vi "resetOutput.vi"(8 "error in (no error)":errorcluster, 11 "K2602 in":refnum<class "K2602.lvclass">) -> (0 "error out":errorcluster, 3 "K2602 out":refnum<class "K2602.lvclass">)   [LabVIEW 2011, in "Hardware.lvlib" / "Channels.lvlib" / "K2602.lvclass"]
uses:
  K2602.lvclass
  AnalogOutput.lvclass
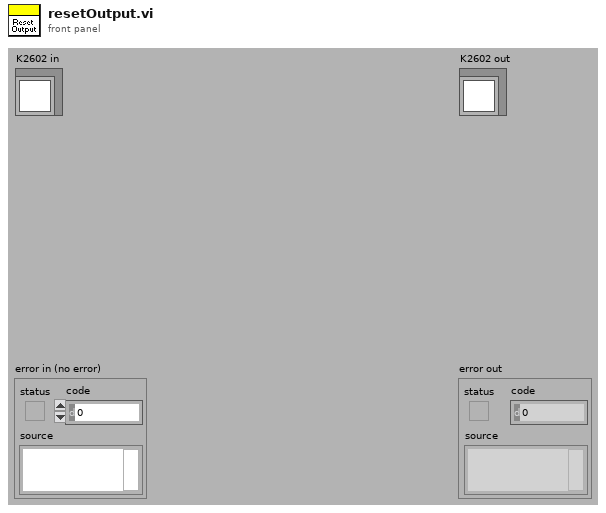
[diagram p1: front panel]
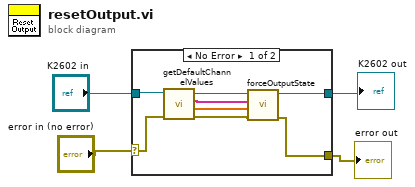
[diagram p0: block diagram]
diagram:
  n1 = case shown="No Error" "error in (no error)" {
    selector: "error in (no error)" -> [w12 w13]
    tunnel: [w8 w14] -> w4
    tunnel: "K2602 in" -> [w11 w14]
    tunnel: [w5 w13] -> w1
    frame No Error {
      n2 = call "getDefaultChannelValues.vi"("error in (no error)"=w12, "AnalogOutput in"=w11) -> ("error out"=w10:errorcluster, "calibratedValues"=w6:dbl[], "channel_addresses"=w7:string[], "AnalogOutput out"=w9:refnum<class "K2602.lvclass">)  [unwired: 6 in]
      n3 = call-dynamic "forceOutputState.vi"("error in (no error)"=w10, "calibratedValues"=w6, "channel_addresses"=w7, "K2602 in"=w9) -> ("error out"=w5:errorcluster, "K2602 out"=w8:refnum<class "K2602.lvclass">)  [unwired: 6 in]
    }
    frame Error {
    }
  }
  "error out" <- w1
  "K2602 out" <- w4
